vi "const_cluster_spymessage.vi"() -> (0 "SpyMessage{}":T1 {"AckBytes [8]" format="%.0x"; "Data [8]" format="%.0x"; "ArbIDOrHeader" format="%.0x"; "DescriptionID" format="%.0x"; "NetworkID" format="%.0x"})   [LabVIEW 2009]
uses:
  ctl spymessage.ctl
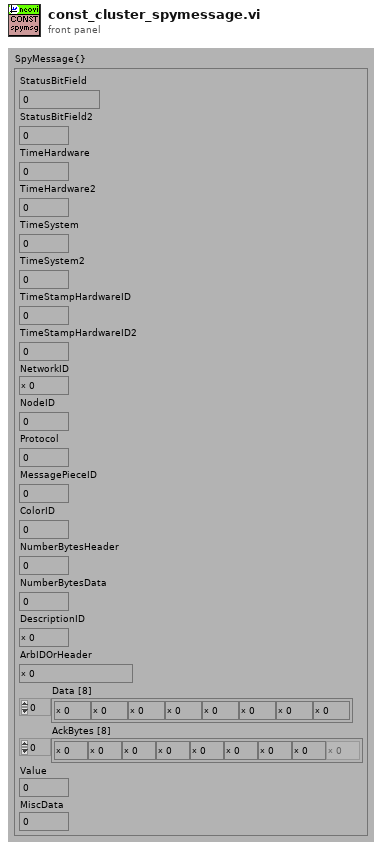
[diagram p1: front panel]
types:
  T1 = typedef "ctl spymessage.ctl" = cluster{"StatusBitField":u32, "StatusBitField2":u32, "TimeHardware":u32, "TimeHardware2":u32, "TimeSystem":u32, "TimeSystem2":u32, "TimeStampHardwareID":u8, "TimeStampHardwareID2":u8, "NetworkID":u8, "NodeID":u8, "Protocol":u8, "MessagePieceID":u8, "ColorID":u8, "NumberBytesHeader":u8, "NumberBytesData":u8, "DescriptionID":u16, "ArbIDOrHeader":u32, "Data [8]":u8[], "AckBytes [8]":u8[], "Value":sgl, "MiscData":u8}
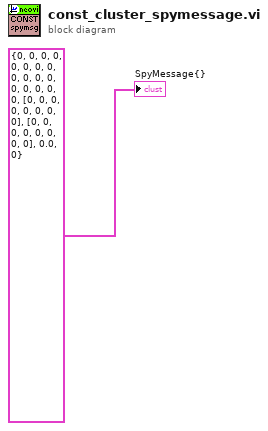
[diagram p0: block diagram]
diagram:
  "SpyMessage{}" <- T1 {"StatusBitField"=0, "StatusBitField2"=0, "TimeHardware"=0, "TimeHardware2"=0, "TimeSystem"=0, "TimeSystem2"=0, "TimeStampHardwareID"=0, "TimeStampHardwareID2"=0, "NetworkID"=0, "NodeID"=0, "Protocol"=0, "MessagePieceID"=0, "ColorID"=0, "NumberBytesHeader"=0, "NumberBytesData"=0, "DescriptionID"=0, "ArbIDOrHeader"=0, "Data [8]"=[0, 0, 0, 0, 0, 0, 0, 0], "AckBytes [8]"=[0, 0, 0, 0, 0, 0, 0, 0], "Value"=0.0, "MiscData"=0} ("SpyMessage{}")
